vi "Receive.vi"(8 "error in (no error)":errorcluster, 11 "Tovey9150 in":refnum<class "Tovey 9150.lvclass">) -> (0 "error out":errorcluster, 2 "Response":string, 3 "Tovey9150 out":refnum<class "Tovey 9150.lvclass">)   [LabVIEW 2015, in "Tovey 9150.lvclass"]
uses:
  Tovey 9150.lvclass
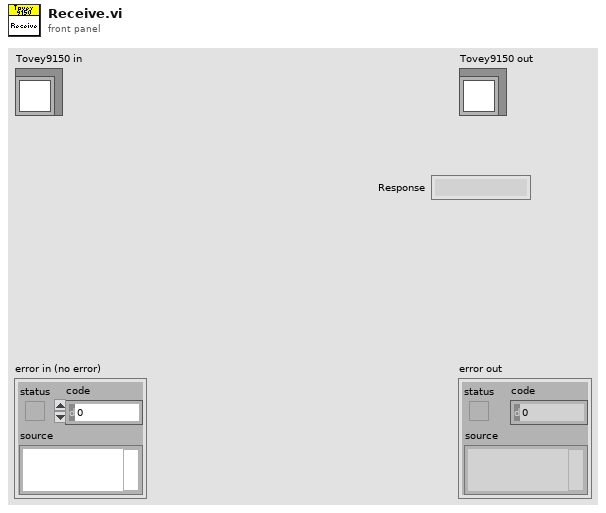
[diagram p1: front panel]
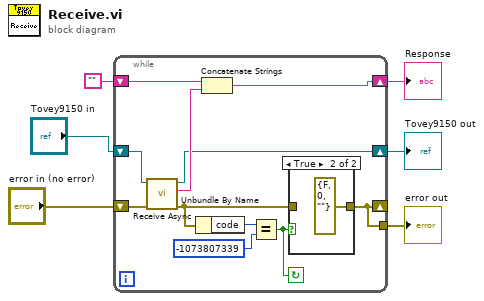
[diagram p0: block diagram]
diagram:
  n1 = while {
    shift-right: [w11] -> w3
    shift-left: "Tovey9150 in" -> [w17]
    shift-right: [w7] -> _
    shift-left: "error in (no error)" -> [w16]
    shift-right: [w12] -> w2
    shift-left: "" -> [w10]
    tunnel: [w7] -> w1
    stop <- w9 continue-if-true
    n2 = call "Receive Async.vi"("error in (no error)"=w16, "Tovey9150 in"=w17) -> ("error out"=w8:errorcluster, "Response"=w13:string, "Tovey9150 out"=w11:refnum<class "Tovey 9150.lvclass">)  [unwired: 7 in]
    n3 = Unbundle By Name(w8) -> ("code"=w14:i32)
    n4 = Concatenate Strings(w10, w13) -> (w12:string)
    n5 = Equal?(x=w14, y=-1073807339) -> (x = y?=w9:bool)
    n6 = case shown="True" w9 {
      tunnel: [w18 errorcluster {"status"=FALSE, "code"=0, "source"=""} ("error out")] -> w7
      tunnel: w8 -> [w18 _]
      frame False {
      }
      frame True {
      }
    }
  }
  "error out" <- w1
  "Tovey9150 out" <- w3
  "Response" <- w2
